vi "Debug - Mid Level - Logging Tool.vi"(8 "Error In":errorcluster, 11 "DTACQ Connection Data In":T1={"Description"="", "Address"="", "Port"=0, "timeout (ms)"=5000, "Termination Character"="\n", "TCP Connection Reference"=refnum, "Open Connection"=FALSE}) -> (0 "Error Out":errorcluster, 3 "DTACQ Connection Data Out":T1={"Description"="", "Address"="", "Port"=0, "timeout (ms)"=5000, "Termination Character"="\n", "TCP Connection Reference"=refnum, "Open Connection"=FALSE})   [LabVIEW 2017, in "Communications Library.lvlib"]
doc: "Adds information to the debug log, every time the error handler is called.\n\nEnable this VI, by setting VERBOSE_DEBUG==TRUE \n(right click on the project in project explorer, select properties, select conditional disable symbols, add VERBOSE_DEBUG and set Value to TRUE)\n\nNote: The error handler is called, regardless of the error state, causing this VI to create a log at the conclussion of every method call at the Mid-Level driver layer."
uses:
  Communications Library.lvlib
  Typedefs/DTACQ Connection Data--Cluster.ctl
  Typedefs/Debug - TCP Write Type--Enum.ctl
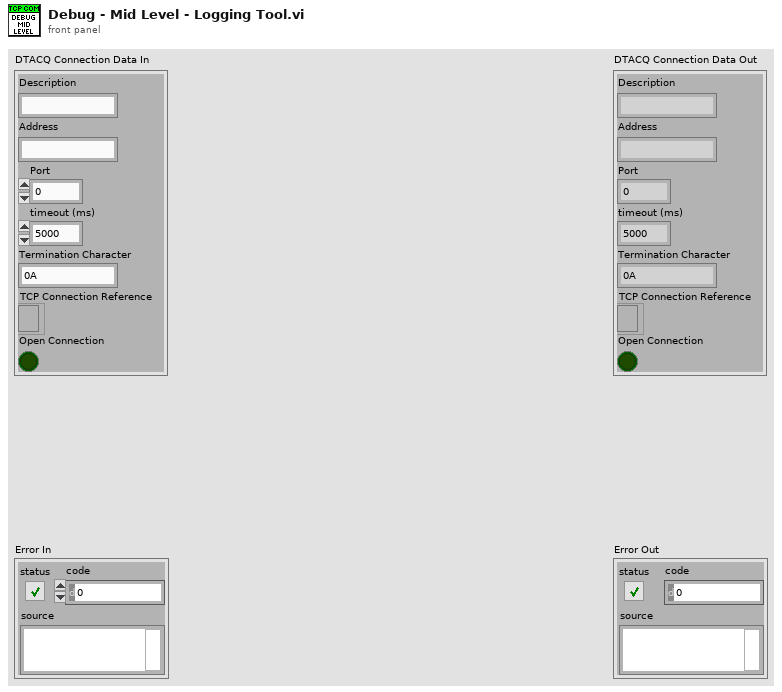
[diagram p1: front panel]
types:
  T1 = typedef "Communications Library.lvlib/DTACQ Connection Data--Cluster.ctl" = cluster{"Description":string, "Address":string, "Port":u16, "timeout (ms)":i32, "Termination Character":string, "TCP Connection Reference":refnum<k5>, "Open Connection":bool}
  T2 = typedef "Communications Library.lvlib/Debug - TCP Write Type--Enum.ctl" = enum16{"Log IP and Port Number", "Append New Line"}
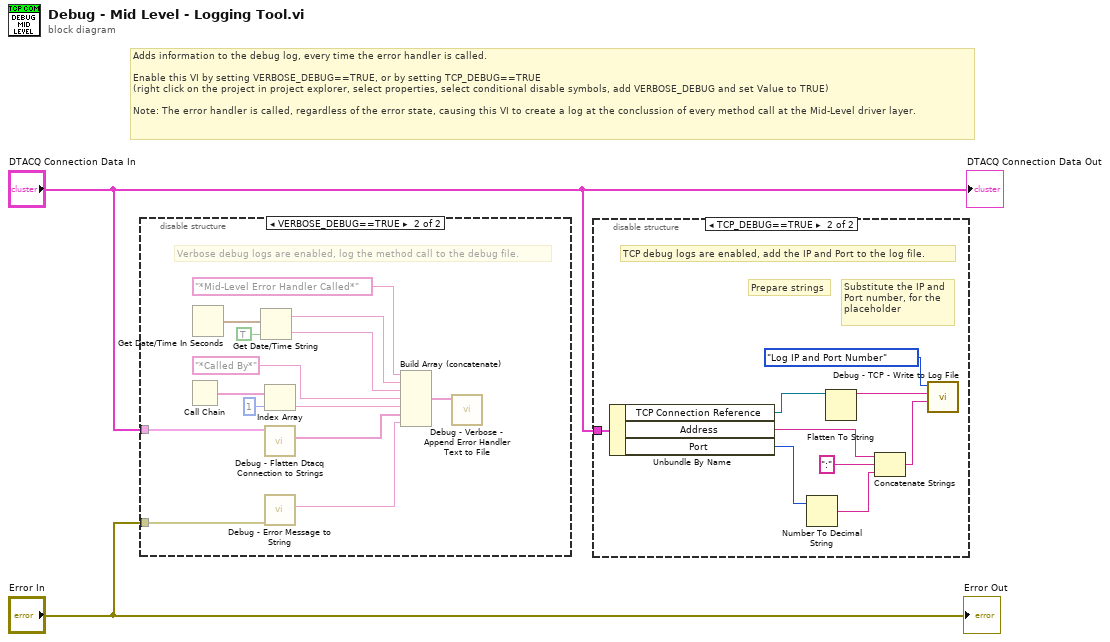
[diagram p0: block diagram]
diagram:
  # "Adds information to the debug log, every time the error handler is called.\n\nEnable this VI by setting VERBOSE_DEBUG==TRUE, or by setting TCP_DEBUG==TRUE\n(right click on the project in project explorer, select properties, select conditional disable symbols, add VERBOSE_DEBUG and set Value to TRUE)\n\nNote: The error handler is called, regardless of the error state, causing this VI to create a log at the conclussion of every method call at the Mid-Level driver layer."
  n1 = disable-structure shown="VERBOSE_DEBUG==TRUE" {
    disable-tunnel: "Error In" -> [_ w6]
    disable-tunnel: "DTACQ Connection Data In" -> [_ w5]
    frame condition #0 (active) {
    }
    frame condition #1 {
      # "Verbose debug logs are enabled, log the method call to the debug file."
      n2 = Call Chain() -> (call chain=w12:string[])
      n3 = Get Date/Time In Seconds() -> (seconds since 1Jan1904=w11:timestamp)
      n4 = Get Date/Time String(seconds (now)=w11, want seconds? (F)=TRUE) -> (date string=w13:string, time string=w14:string)  [unwired: 1 in]
      n5 = Index Array(array=w12, index=1) -> (element=w15:string)
      n6 = call "Debug - Flatten Dtacq Connection to Strings.vi"("DTACQ Connection Data In"=w5) -> ("Array of Strings"=w4:string[])  [unwired: 10 in]
      n7 = call "Debug - Error Message to String.vi"("error in"=w6) -> ("Error Message"=w3:string)  [unwired: 9 in, 1 out]
      n8 = Build Array (concatenate)("*Mid-Level Error Handler Called*", w13, w14, "*Called By*", w15, w4, w3) -> (w16:string[])
      n9 = call "Debug - Verbose - Append Error Handler Text to File.vi"("Strings to Append"=w16) -> ()  [unwired: 11 in]
    }
  }
  n10 = disable-structure shown="TCP_DEBUG==TRUE" {
    disable-tunnel: "DTACQ Connection Data In" -> [_ w25]
    frame condition #0 {
    }
    frame condition #1 (active) {
      # "Substitute the IP and\nPort number, for the\nplaceholder"
      # "Prepare strings"
      # "TCP debug logs are enabled, add the IP and Port to the log file."
      n11 = Unbundle By Name(w25) -> ("TCP Connection Reference"=w24:refnum<k5>, "Address"=w22:string, "Port"=w23:u16)
      n12 = Number To Decimal String(number=w23) -> (decimal integer string=w20:string)  [unwired: 1 in]
      n13 = Flatten To String(anything=w24) -> (data string=w18:string)  [unwired: 3 in, 2 out]
      n14 = Concatenate Strings(w22, ":" ("string"), w20) -> (w19:string)
      n15 = call "Debug - TCP - Write to Log File.vi"("Transmission Log (or IP and Port String)"=w19, "Flattened TCP Reference"=w18, "Type of Write Opperation"=Debug_-_TCP_Write_Type--Enum."Log IP and Port Number") -> ()  [unwired: 9 in]
    }
  }
  "Error Out" <- "Error In"
  "DTACQ Connection Data Out" <- "DTACQ Connection Data In"
